vi "execute_initial_value_policy.vi"(8 "error in (no error)":errorcluster, 9 "Last Publish Time":timestamp, 10 "Last Topic Value":variant, 11 "TimedAverageSubscription In":refnum<class "TimedAverageSubscription.lvclass">) -> (0 "error out":errorcluster, 3 "TimedAverageSubscription Out":refnum<class "TimedAverageSubscription.lvclass">)   [LabVIEW 2017, in "SubscriptionPolicy.lvlib" / "TimedAverageSubscription.lvclass"]
uses:
  TimedAverageSubscription.lvclass
  TimedAverageSubscription.lvclass/TimedAverageSubscription.ctl
  <vilib>/Composed Systems/Timed Average Buffer/TimedAverageBuffer.lvclass/TimedAverageBuffer.ctl
  <vilib>/Utility/High Resolution Relative Seconds.vi
  <vilib>/Composed Systems/Timed Average Buffer/TimedAverageBuffer.lvclass
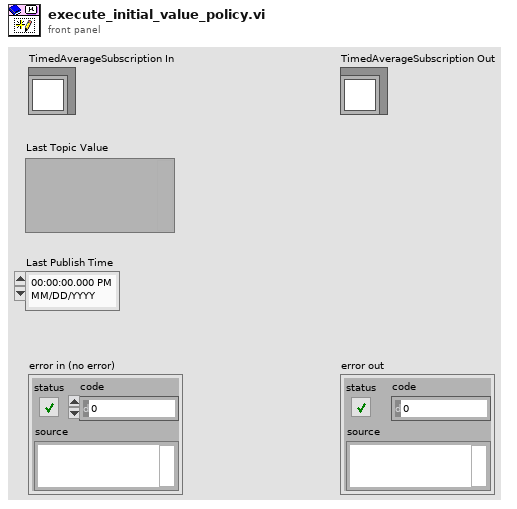
[diagram p1: front panel]
types:
  T1 = typedef "TimedAverageBuffer.lvlib/TimedAverageBuffer.lvclass/TimedAverageBuffer Reference.ctl" = refnum<data-value>
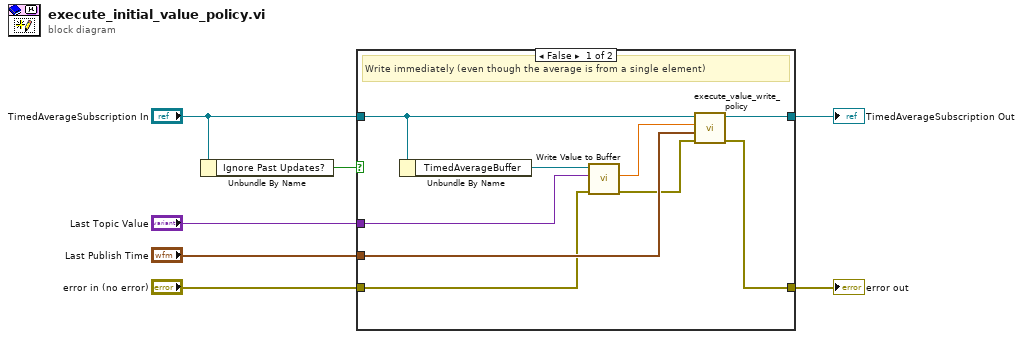
[diagram p0: block diagram]
diagram:
  n1 = Unbundle By Name("TimedAverageSubscription In") -> ("Ignore Past Updates?"=w5:bool)
  n2 = case shown="False" w5 {
    tunnel: "TimedAverageSubscription In" -> [w13 w18]
    tunnel: [w16 w18] -> w6
    tunnel: "Last Topic Value" -> [w11 _]
    tunnel: "Last Publish Time" -> [w15 _]
    tunnel: "error in (no error)" -> [w10 w17]
    tunnel: [w14 w17] -> w1
    frame False {
      # "Write immediately (even though the average is from a single element)"
      n3 = Unbundle By Name(w13) -> ("TimedAverageBuffer"=w12:T1)
      n4 = call <vilib>:"Write Value to Buffer.vi"("error in (no error)"=w10, "Value"=w11, "Timed Average Buffer"=w12) -> ("error out"=w9:errorcluster, "Average"=w8:dbl)  [unwired: 5 in, 2 out]
      n5 = call-dynamic "execute_value_write_policy.vi"("error in (no error)"=w9, "Publish Time"=w15, "New Topic Value"=w8, "TimedAverageSubscription In"=w13) -> ("error out"=w14:errorcluster, "TimedAverageSubscription Out"=w16:refnum<class "TimedAverageSubscription.lvclass">)  [unwired: 6 in]
    }
    frame True {
      # "Ignore past updates"
    }
  }
  "error out" <- w1
  "TimedAverageSubscription Out" <- w6
